vi "Acquire.vi"(8 "error in (no error)":errorcluster, 9 "minimum value":dbl=-5.0, 10 "maximum value":dbl=5.0, 11 "physical channels":refnum<k21>) -> (0 "error out":errorcluster, 2 "Graph Data":waveform(dbl)[](array[waveform]))   [LabVIEW 2020, in "Acquisition.lvlib"]
doc: "Perform the acquisition. Replace the contents of this diagram with calls to acquisition hardware.\n_____\nBased on Delacor QMH Project Template 5.0.0.82."
uses:
  Acquisition.lvlib
  <vilib>/ULx/Create Channel.llb/ULx Create Channel (AI-Voltage-Basic).vi
  <vilib>/ULx/Timing.llb/ULx Timing (Sample Clock).vi
  <vilib>/ULx/Read.llb/ULx Read (Analog Wfm 1Chan NSamp).vi
  <vilib>/express/express shared/ex_Modify Signal Name.vi
  <vilib>/express/express arith-compare/Formula/XNode/ExpressFormulaBlockNode.xnode
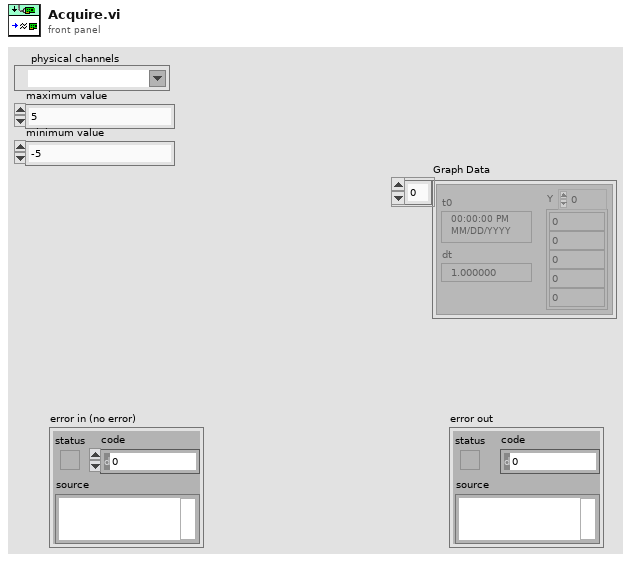
[diagram p1: front panel]
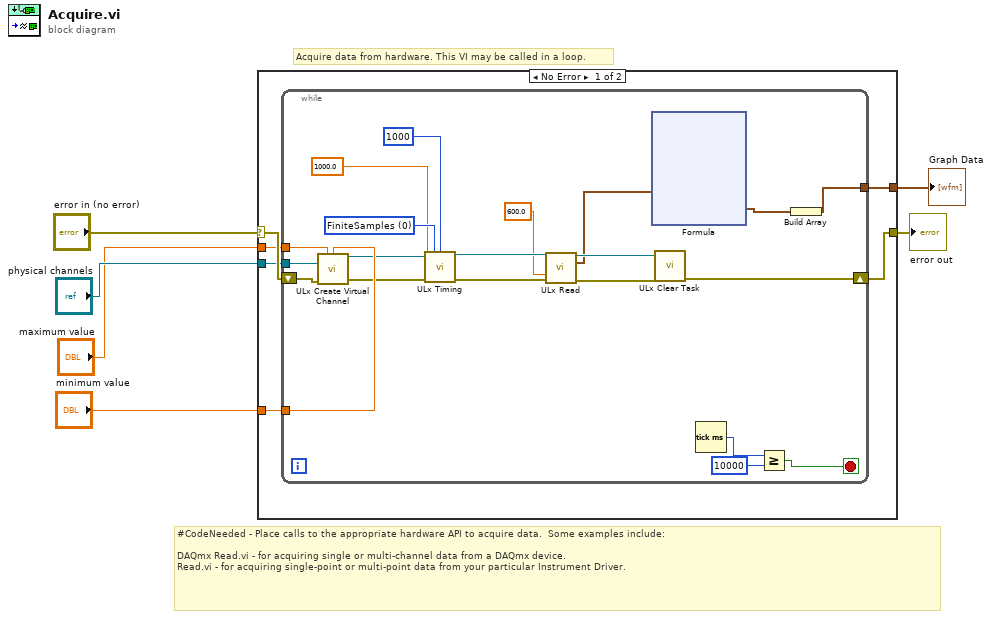
[diagram p0: block diagram]
diagram:
  # "Acquire data from hardware. This VI may be called in a loop."
  # "#CodeNeeded - Place calls to the appropriate hardware API to acquire data.  Some examples include:\n\nDAQmx Read.vi - for acquiring single or multi-channel data from a DAQmx device.\nRead.vi - for acquiring single-point or multi-point data from your particular Instrument Driver."
  n1 = case shown="No Error" "error in (no error)" {
    selector: "error in (no error)" -> [w12 w48]
    tunnel: [w8 w48] -> w5
    tunnel: "physical channels" -> [w11 _]
    tunnel: "maximum value" -> [w10 _]
    tunnel: "minimum value" -> [w9 _]
    tunnel: [w7 _] -> w1
    frame No Error {
      n2 = while {
        tunnel: w11 -> [w32]
        tunnel: w10 -> [w31]
        tunnel: w9 -> [w30]
        tunnel: [w17] -> w7
        shift-right: [w18] -> w8
        shift-left: w12 -> [w33]
        stop <- w15 stop-if-true
        w27 = 0 items=["FiniteSamples", "ContinuousSamples"] ("sample mode")
        n3 = call-poly <vilib>:"ULx Create Virtual Channel.vi"("maximum value"=w31, "minimum value"=w30, "physical channels"=w32, "error in"=w33) -> ("task out"=w28:refnum<k24>, "error out"=w29:errorcluster)  [unwired: 10 in]
        n4 = call-poly <vilib>:"ULx Timing.vi"("task in"=w28, "sample mode"=w27, "samples per channel"=1000, "rate"=1000.0, "error in"=w29) -> ("task out"=w24:refnum<k24>, "error out"=w25:errorcluster)  [unwired: 9 in]
        n5 = call-poly <vilib>:"ULx Read.vi"("task in"=w24, "timeout"=600.0, "error in"=w25) -> ("task out"=w21:refnum<k24>, "data"=w20:waveform(dbl), "error out"=w22:errorcluster)  [unwired: 10 in]
        n6 = xnode "Formula"("X1"=w20) -> ("Result"=w19:waveform(dbl))  [unwired: 1 in, 1 out]
        n7 = call <vilib>:"ULx Clear Task.vi"("task in"=w21, "error in"=w22) -> ("error out"=w18:errorcluster)  [unwired: 13 in]
        n8 = Tick Count (ms)() -> (millisecond timer value=w14:u32)
        n9 = Greater Or Equal?(x=w14, y=u32 10000) -> (x >= y?=w15:bool)
        n10 = Build Array(w19) -> (w17:waveform(dbl)[])
      }
    }
    frame Error {
    }
  }
  "error out" <- w5
  "Graph Data" <- w1
